vi "6.3.1.vi"() -> ()   [LabVIEW 2018]
panel:
  out "웨이브폼 차트":dbl(graph)
  in  "경로":path
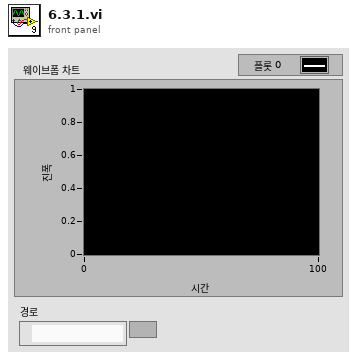
[diagram p1: front panel]
types:
  T1 = enum16{"open", "replace", "create", "open or create", "replace or create", "replace or create with confirmation"}
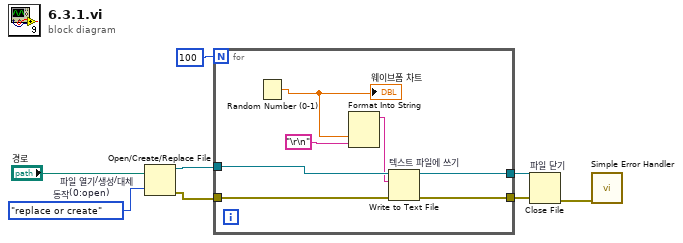
[diagram p0: block diagram]
diagram:
  w7 = T1."replace or create"  # 동작(0:open)
  n1 = Open/Create/Replace File "파일 열기/생성/대체"(file path (use dialog)="경로", operation (0:open)=w7) -> (refnum out=w4:refnum<file>, error out=w1:errorcluster)  [unwired: 4 in, 1 out]
  n2 = for {
    N: 100 -> [_]
    tunnel: w4 -> [w15]
    tunnel: [w14] -> w3
    tunnel: [w13] -> w2
    tunnel: w1 -> [w12]
    n3 = Random Number (0-1)() -> (number: 0 to 1=w11:dbl)
    "웨이브폼 차트" <- w11
    n4 = Format Into String(w11, "\r\n") -> (resulting string=w9:string)  [unwired: 3 in, 1 out]
    n5 = Write to Text File "텍스트 파일에 쓰기"(file (use dialog)=w15, text=w9, error in=w12) -> (refnum out=w14:refnum<file>, error out=w13:errorcluster)  [unwired: 1 in, 1 out]
  }
  n6 = Close File "파일 닫기"(refnum=w3, error in=w2) -> (error out=w6:errorcluster)  [unwired: 1 out]
  n7 = call <vilib>:"Simple Error Handler.vi"("error in (no error)"=w6) -> ()  [unwired: 4 in, 5 out]
